vi "getHPs.vi"(11 "ILCCommunications in":refnum<class "ILCCommunications.lvclass">) -> (2 "HPs":refnum<class "HPILC.lvclass">[](array[class]), 3 "ILCCommunications out":refnum<class "ILCCommunications.lvclass">)   [LabVIEW 2016, in "ILCCommunications.lvclass"]
uses:
  ILCCommunications.lvclass
  Common_RT_HPILC/HPILC/HPILC.lvclass
  ILCCommunications.lvclass/ILCCommunications.ctl
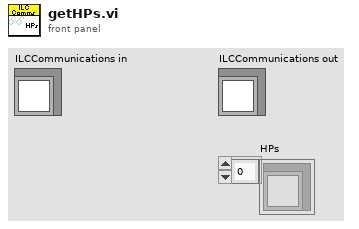
[diagram p1: front panel]
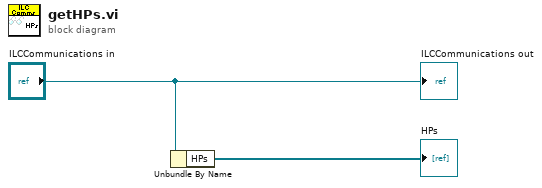
[diagram p0: block diagram]
diagram:
  n1 = Unbundle By Name("ILCCommunications in") -> ("HPs"=→"HPs":refnum<class "HPILC.lvclass">[])
  "ILCCommunications out" <- "ILCCommunications in"
